vi "enumerateStaticDependencies.vi"(8 "error in (no error)":errorcluster, 11 "Microscope":refnum<class "Microscope.lvclass">) -> (0 "error out":errorcluster, 2 "Static Dependencies":refnum<class "Dependency.lvclass">[](array[class]), 3 "Microscope out":refnum<class "Microscope.lvclass">)   [LabVIEW 2020, in "Microscope.lvclass"]
doc: "JKI State Machine Objects (SMO) 1.1.0.20\nJKI - JKI\nCopyright (c) 2016, JKI"
uses:
  Microscope.lvclass
  <vilib>/JKI/JKI SMO/Dependency/Dependency.lvclass
  Typedefs/Dependencies--Cluster.ctl
  XYStage/XYStage.lvclass
  C:/Program Files/National Instruments/LabVIEW 2020/vi.lib/JKI/JKI SMO/SMO/SMO.lvclass
  Camera/Camera.lvclass
  <vilib>/JKI/JKI SMO/SMO/SMO.lvclass
  Microscope.lvclass/Microscope.ctl
panel:
  # "For instructions on how to use the JKI State Machine Objects, examples and video tutorials, visit:\nhttp://jki.net/state-machine-objects/\n\nJKI State Machine Objects™\nhttp://jki.net/state-machine-objects/\nCopyright (C) 2005-2015, JKI <info@jki.net>\nALL RIGHTS RESERVED"
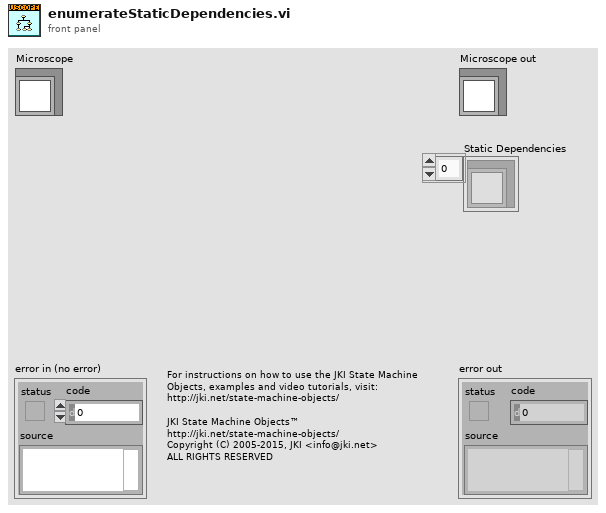
[diagram p1: front panel]
types:
  T1 = typedef "Microscope.lvclass/Dependencies--Cluster.ctl" = cluster{"XYStage":refnum<class "XYStage.lvclass">, "Camera":refnum<class "Camera.lvclass">}
  T2 = typedef "Microscope.lvclass/Configuration--Cluster.ctl" = cluster{"XY Stage":string, "Camera":string, "image output folder":path, "filetype":string}
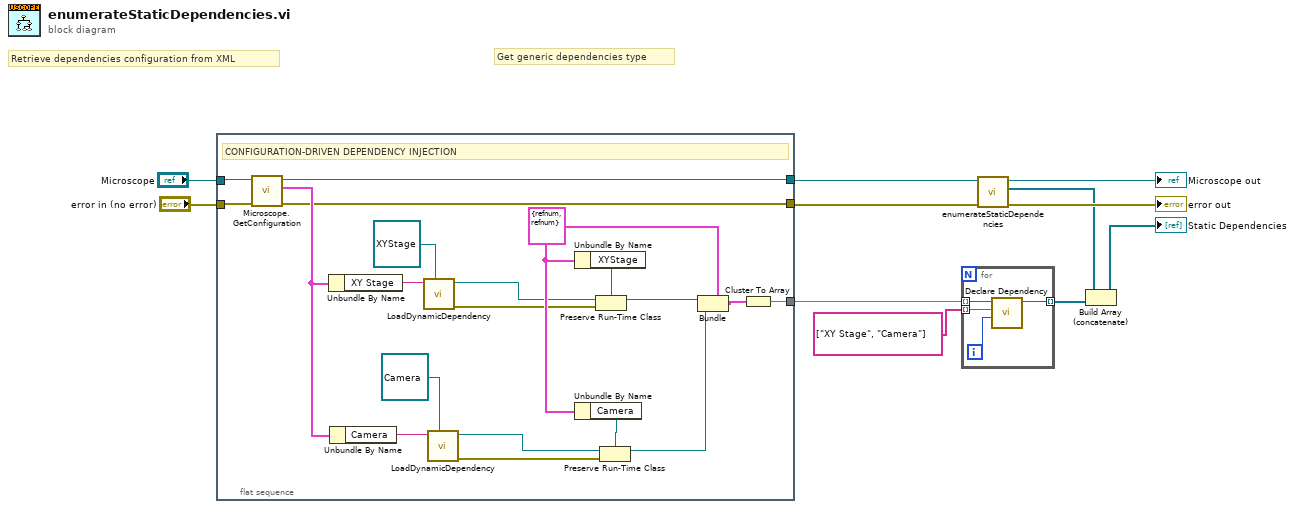
[diagram p0: block diagram]
diagram:
  # "Get generic dependencies type"
  # "Retrieve dependencies configuration from XML"
  n1 = flat-sequence {
    tunnel: "Microscope" -> [w31]
    tunnel: "error in (no error)" -> [w13]
    tunnel: [w28] -> w4
    tunnel: [w12] -> w3
    tunnel: [w24] -> w2
    frame #0 {
      w26 = T1 {"XYStage"=refnum, "Camera"=refnum} ("Dependencies")
      # "CONFIGURATION-DRIVEN DEPENDENCY INJECTION"
      n2 = call "Microscope.GetConfiguration.vi"("error in (no error)"=w13, "Microscope"=w31) -> ("error out"=w12:errorcluster, "Configuration"=w30:T2, "Microscope out"=w28:refnum<class "Microscope.lvclass">)  [unwired: 7 in]
      n3 = Unbundle By Name(w30) -> ("XY Stage"=w16:string)
      n4 = Unbundle By Name(w30) -> ("Camera"=w21:string)
      n5 = call "LoadDynamicDependency.vi"("SMO in"=refnum<class "XYStage.lvclass"> refnum ("XYStage.lvclass"), "Camera"=w16) -> ("error out"=w15:errorcluster, "SMO out"=w14:refnum<class "XYStage.lvclass">)  [unwired: 8 in]
      n6 = call "LoadDynamicDependency.vi"("SMO in"=refnum<class "Camera.lvclass"> refnum ("Camera.lvclass"), "Camera"=w21) -> ("error out"=w18:errorcluster, "SMO out"=w20:refnum<class "Camera.lvclass">)  [unwired: 8 in]
      n7 = Unbundle By Name(w26) -> ("XYStage"=w27:refnum<class "XYStage.lvclass">)
      n8 = Unbundle By Name(w26) -> ("Camera"=w29:refnum<class "Camera.lvclass">)
      n9 = Preserve Run-Time Class(object in=w14, error in=w15, 2:w27) -> (object out=w23:refnum<class "XYStage.lvclass">)  [unwired: 1 out]
      n10 = Preserve Run-Time Class(object in=w20, error in=w18, 2:w29) -> (object out=w22:refnum<class "Camera.lvclass">)  [unwired: 1 out]
      n11 = Bundle(cluster=w26, "XYStage"=w23, "Camera"=w22) -> (w25:T1)
      n12 = Cluster To Array(cluster=w25) -> (array=w24:refnum<class "SMO.lvclass">[])
    }
  }
  n13 = for {
    tunnel: [w35] -> w9 mode=indexing
    tunnel: w2 -> [w34] mode=indexing
    tunnel: string[] ["XY Stage", "Camera"] -> [w32] mode=indexing
    i -> [w33]
    n14 = call <vilib>:"Declare Dependency.vi"("Start Order (0)"=w33, "Name"=w32, "Type"=w34) -> ("Dependency out"=w35:refnum<class "Dependency.lvclass">)  [unwired: 7 in, 1 out]
  }
  n15 = call-parent "enumerateStaticDependencies.vi"("error in (no error)"=w3, "SMO"=w4) -> ("error out"=→"error out":errorcluster, "Static Dependencies"=w7:refnum<class "Dependency.lvclass">[], "SMO out"=→"Microscope out":refnum<class "Microscope.lvclass">)  [unwired: 7 in]
  n16 = Build Array (concatenate)(w7, w9) -> (→"Static Dependencies":refnum<class "Dependency.lvclass">[])
